vi "Remove Tildes (String).vi"(3 "String In":string) -> (1 "String Out":string)   [LabVIEW 2019]
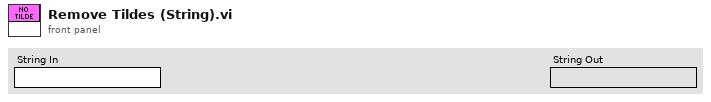
[diagram p1: front panel]
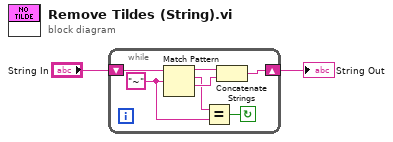
[diagram p0: block diagram]
diagram:
  n1 = while {
    shift-right: [w6] -> w1
    shift-left: "String In" -> [w9]
    stop <- w3 continue-if-true
    w5 = "~" ("regular expression")
    n2 = Match Pattern(string=w9, regular expression=w5) -> (before substring=w8:string, match substring=w4:string, after substring=w7:string)  [unwired: 1 in, 1 out]
    n3 = Equal?(x=w4, y=w5) -> (x = y?=w3:bool)
    n4 = Concatenate Strings(w8, w7) -> (w6:string)
  }
  "String Out" <- w1
